vi "SpectrogramExample.vi"() -> ()   [LabVIEW 2014]
doc: "Continuously acquires a communication signal that starts immediately. The device is not synchronized to external Reference Clocks or timebases."
uses:
  <vilib>/measure/NI_MAPro.lvlib
  <vilib>/measure/maspectr.llb/FFT Power Spectrum for 1 Chan (CDB).vi
  <instrlib>/niUSRP/niUSRP Fetch Rx Data (CDB WDT).vi
panel:
  in  "device names":refnum<k15>
  in  "Update Rate (s)":dbl=0.1 min=0.001 step=0.025
  in  "Dynamic Range (dB)":cluster{dbl, dbl}(slide)={0.09852216748768905, -121.37931034482759} scale=-140.0..40.0
  in  "Waterfall Time Scale (s)":i32=5
  out "Waterfall Plot":dbl[][](graph)
  in  "enabled channel":string(combo)="0"
  in  "stop":bool
  in  "active antenna":string="RX1"
  in  "timeout":dbl=10.0 format="%#.3ps"
  in  "number of samples":i64=16384
  out "error out":errorcluster
  out "coerced gain":dbl format="%#_6f"
  out "coerced carrier frequency":dbl=100000.0 format="%#_6p"
  out "coerced IQ rate [S/sec]":dbl=100000.0 format="%#_6p"
  in  "gain":dbl=1.0 format="%#_6f"
  in  "carrier frequency":dbl=2000000000.0 format="%#_6p"
  in  "IQ rate [S/sec]":dbl=1000000.0 format="%#_6p"
  # "Radio Controls"
  # "Graph Controls"
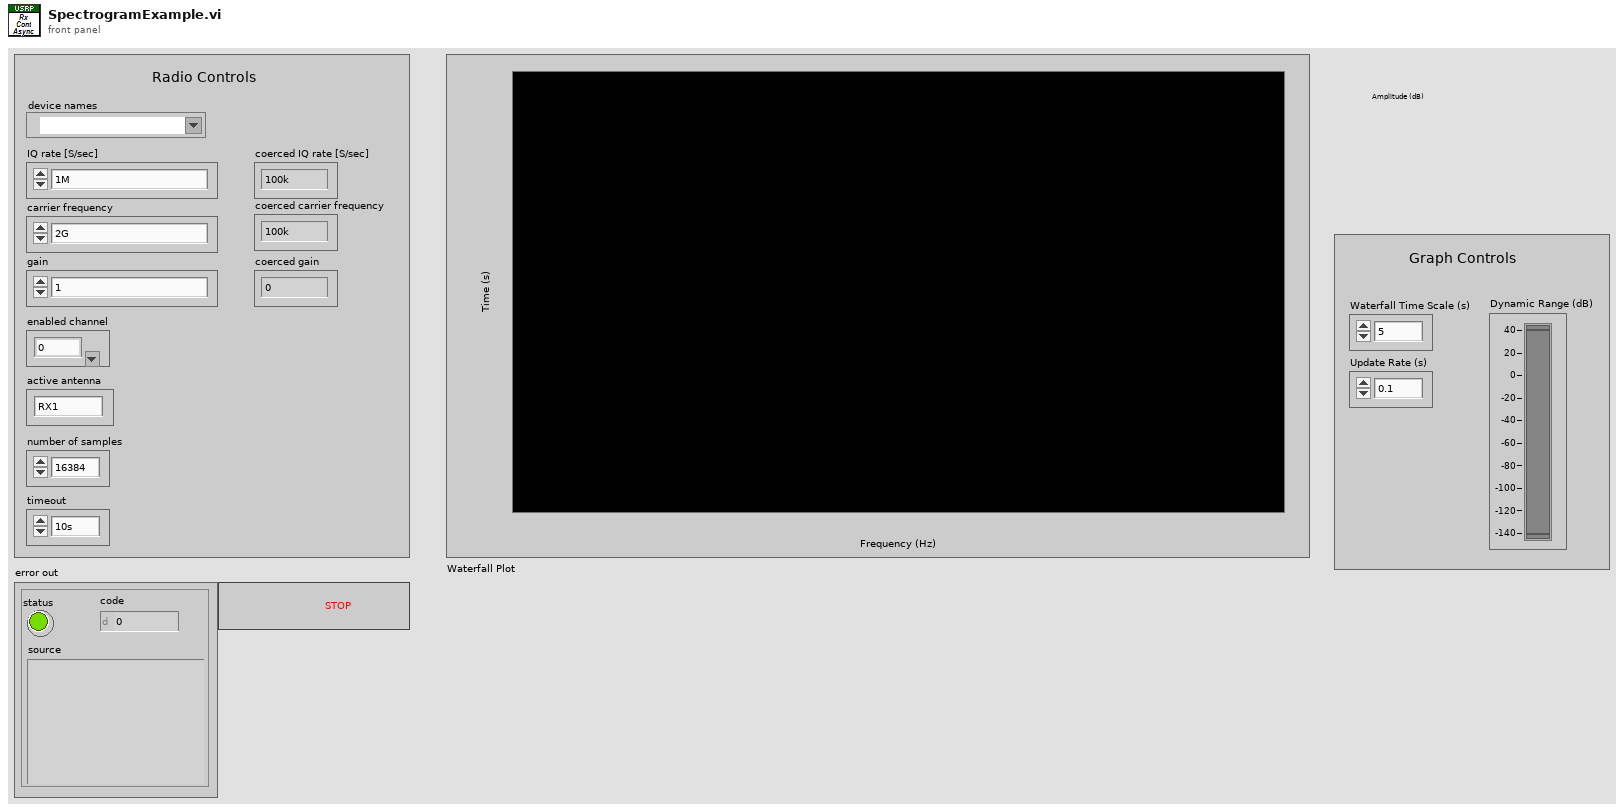
[diagram p1: front panel]
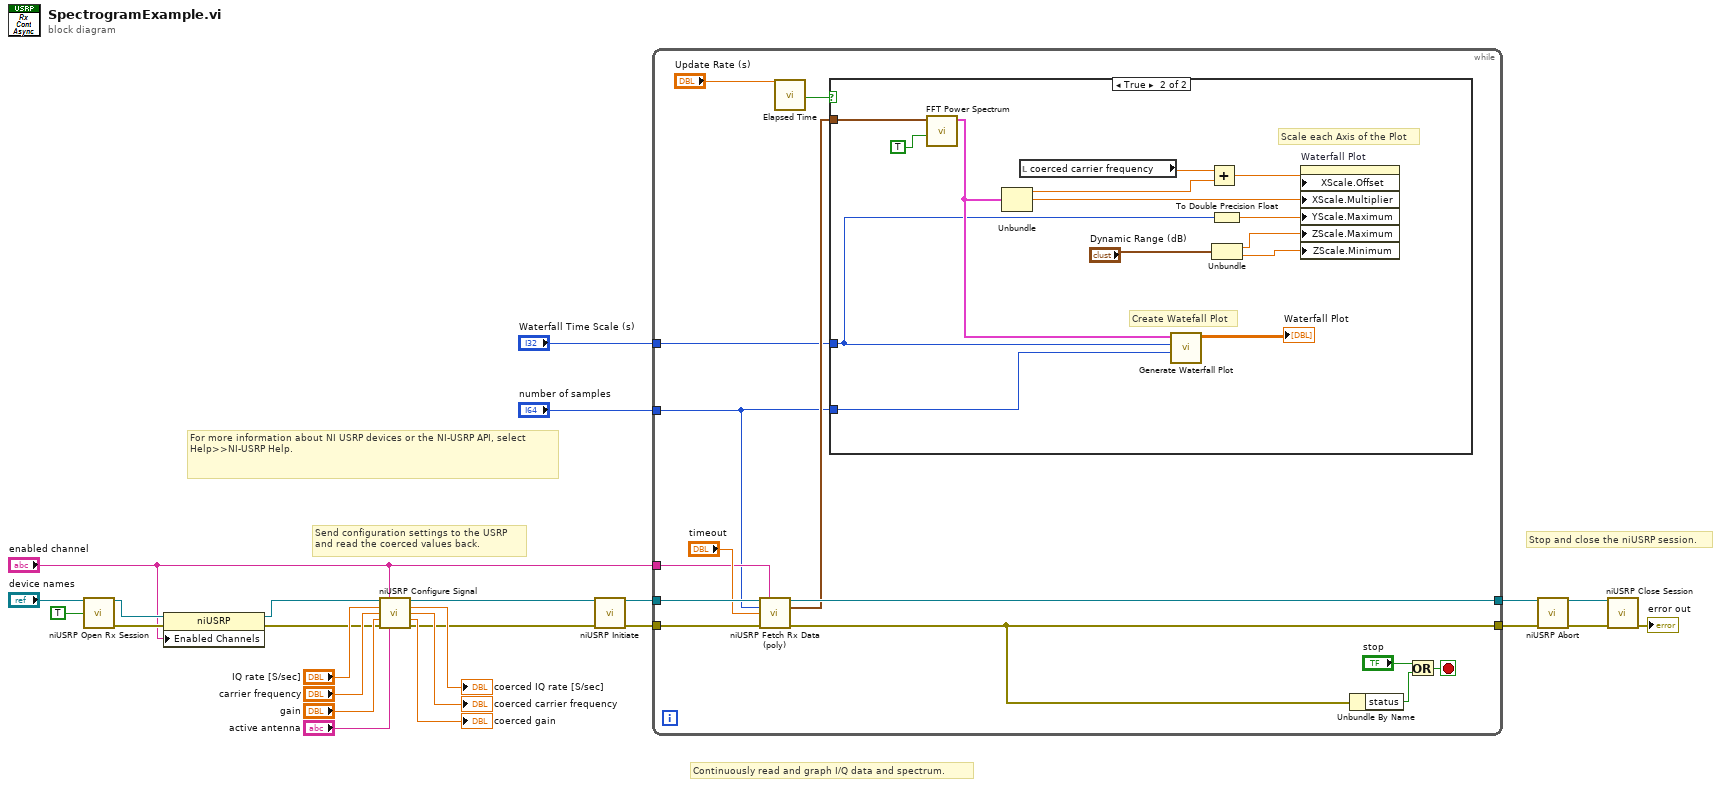
[diagram p0: block diagram]
diagram:
  # "For more information about NI USRP devices or the NI-USRP API, select Help>>NI-USRP Help."
  # "Stop and close the niUSRP session."
  # "Continuously read and graph I/Q data and spectrum."
  # "Send configuration settings to the USRP\nand read the coerced values back."
  n1 = call <instrlib>:"niUSRP Open Rx Session.vi"("device names"="device names", "reset"=TRUE) -> ("session handle out"=w9:refnum<k15>, "error out"=w7:errorcluster)  [unwired: 12 in]
  n2 = property class="niUSRP"(reference=w9, error in=w7, "Enabled Channels"="enabled channel") -> (reference out=w8:refnum<k15>, error out=w6:errorcluster)
  n3 = call <instrlib>:"niUSRP Configure Signal.vi"("session handle"=w8, "channel list"="enabled channel", "IQ rate"="IQ rate [S/sec]", "carrier frequency"="carrier frequency", "gain"="gain", "error in (no error)"=w6, "active antenna"="active antenna") -> ("session handle out"=w11:refnum<k15>, "coerced IQ rate"=→"coerced IQ rate [S/sec]":dbl, "coerced carrier frequency"=→"coerced carrier frequency":dbl, "coerced gain"=→"coerced gain":dbl, "error out"=w10:errorcluster)  [unwired: 4 in]
  n4 = call <instrlib>:"niUSRP Initiate.vi"("session handle"=w11, "error in (no error)"=w10) -> ("session handle out"=w25:refnum<k15>, "error out"=w24:errorcluster)  [unwired: 12 in]
  n5 = while {
    tunnel: w25 -> [w39]
    tunnel: [w36] -> w23
    tunnel: "enabled channel" -> [w31]
    tunnel: w24 -> [w38]
    tunnel: [w35] -> w22
    tunnel: "number of samples" -> [w28]
    tunnel: "Waterfall Time Scale (s)" -> [w26]
    stop <- w34 stop-if-true
    n6 = call-poly <instrlib>:"niUSRP Fetch Rx Data (poly).vi"("session handle"=w39, "channel list"=w31, "number of samples"=w28, "timeout"="timeout", "error in (no error)"=w38) -> ("session handle out"=w36:refnum<k15>, "data"=w29:waveform(cdb), "error out"=w35:errorcluster)  [unwired: 7 in, 1 out]
    n7 = call "Elapsed Time"("Time Target (s)"="Update Rate (s)") -> ("Time has Elapsed"=w30:bool)  [unwired: 11 in, 7 out]
    n8 = case shown="True" w30 {
      tunnel: w29 -> [_ w52]
      tunnel: w28 -> [_ w50]
      tunnel: w26 -> [_ w40]
      frame False {
      }
      frame True {
        # "Create Watefall Plot"
        # "Scale each Axis of the Plot"
        n9 = call-poly <vilib>:"FFT Power Spectrum.vi"("dB On (F)"=TRUE, "time signal"=w52) -> ("power spectrum"=w44:cluster{"f0":dbl, "df":dbl, "magnitude":dbl[]})  [unwired: 6 in, 3 out]
        n10 = Unbundle(w44) -> ("f0"=w43:dbl, "df"=w42:dbl)  [unwired: 1 out]
        n11 = local read "coerced carrier frequency"() -> (w49:dbl)
        n12 = call "Generate Waterfall Plot.vi"("number of samples"=w50, "Waterfall Time Scale (s)"=w40, "power spectrum"=w44) -> ("Waterfall Plot Output"=→"Waterfall Plot":dbl[][])  [unwired: 8 in]
        n13 = Add(x=w49, y=w43) -> (x+y=w48:dbl)
        n14 = To Double Precision Float(number=w40) -> (double precision float=w41:dbl)
        n15 = Unbundle("Dynamic Range (dB)") -> (w46:dbl, w45:dbl)
        n16 = property on="Waterfall Plot" class="IntGraph (strict)"("XScale.Offset"=w48, "XScale.Multiplier"=w42, "YScale.Maximum"=w41, "ZScale.Maximum"=w46, "ZScale.Minimum"=w45) -> ()  [unwired: 2 in, 2 out]
      }
    }
    n17 = Unbundle By Name(w35) -> ("status"=w32:bool)
    n18 = Or(x="stop", y=w32) -> (x .or. y?=w34:bool)
  }
  n19 = call <instrlib>:"niUSRP Abort.vi"("session handle"=w23, "error in (no error)"=w22) -> ("session handle out"=w20:refnum<k15>, "error out"=w21:errorcluster)  [unwired: 12 in]
  n20 = call <instrlib>:"niUSRP Close Session.vi"("session handle"=w20, "error in (no error)"=w21) -> ("error out"=→"error out":errorcluster)  [unwired: 13 in]
